vi "Event handler-Time series.vi"() -> (0 "error out":errorcluster)   [LabVIEW 2017]
uses:
  Typedefs/Read Write Enum.ctl
  Global Variables/General Globals.vi
  Global Variables/gl_UI Ctrl Refs.vi
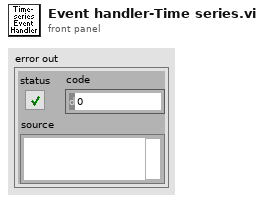
[diagram p1: front panel]
types:
  T1 = enum8{"Enabled", "Disabled", "Disabled and Grayed Out"}
  T2 = typedef "Read Write Enum.ctl" = enum16{"Read", "Write"}
  T3 = typedef "UI ctrl refs cluster.ctl" = cluster{"Top level VI path":path, "Top level VI ref":refnum<vi>, "User menu ref":refnum<k9>, "Sub Panel control":refnum<vi>, "Imaging Param Tab":refnum<vi>, "Occurrence-Start drivers":refnum<k4>, "Occurrence-Speed logging initialised":refnum<k4>, "Occurrence-XYZ stage initialised":refnum<k4>, "Exit button":refnum<vi>, "Status ind":refnum<vi>, "Set as origin":refnum<vi>, "Speed Logging":refnum<vi>, "Time Lapse":refnum<vi>, "Live Imaging":refnum<vi>, "AOL Z Stack":refnum<vi>, "Motor Z Stack":refnum<vi>, "Funct Acq button":refnum<vi>, "Hard Shutter":refnum<vi>, "Virtual Shutter":refnum<vi>, "Laser Power":refnum<vi>, "AOL Mode":refnum<vi>, "Frame Size":refnum<vi>, "Field of View":refnum<vi>, "Dwell Time":refnum<vi>, "Zoom":refnum<vi>, "AOL Z":refnum<vi>, "Objective":refnum<vi>, "Axis":refnum<vi>, "Paths & Names":refnum<vi>, "Experiment folder path (ind.)":refnum<vi>, "Last State (Ind.)":refnum<vi>, "Laser wavelength ind (nm)":refnum<vi>, "Averages":refnum<vi>, "Angle (degrees)":refnum<vi>, "X centre":refnum<vi>, "Y centre":refnum<vi>, "Plane Mode":refnum<vi>, "# Planes":refnum<vi>, "Z Start":refnum<vi>, "Z Stop":refnum<vi>, "Z Step":refnum<vi>, "PMT 1":refnum<vi>, "PMT 2":refnum<vi>, "Stage XYZ Position":refnum<vi>, "Pockels@Z Start":refnum<vi>, "Pockels@Z Stop":refnum<vi>, "Obtain Z Start":refnum<vi>, "Obtain Z Stop":refnum<vi>, "Live stim.trig.period":refnum<vi>, "Live stim.trig.enable":refnum<vi>, "Movement Correction":refnum<vi>, "Load Reference Image":refnum<vi>, "XY Stage Move":refnum<vi>, "MovCor Cluster":refnum<vi>, "RefDAQParam":refnum<vi>, "Funct. Acq. Pockels Modulation":refnum<vi>, "Background MovCor":refnum<vi>, "Ref Laser Power":refnum<vi>, "Enable Video Recording":refnum<vi>, "Video Record-Live Imaging":refnum<vi>, "Video Record-Funct acq":refnum<vi>, "Reference Source":refnum<vi>, "AOL Z-stack Chirps Ready (ind)":refnum<vi>, "Target time between mov.cor. ref triggers (ms)":refnum<vi>, "Funct. Acq. Ref frame save":refnum<vi>, "Tracking button":refnum<vi>, "Show ref plots window":refnum<vi>, "Center freq ind (nm)":refnum<vi>, "Pickup mode (ind)":refnum<vi>, "Logging queue (ind)":refnum<vi>, "Back aperture power (ind.)":refnum<vi>, "Power after objective (ind.)":refnum<vi>, "Switch user":refnum<vi>}
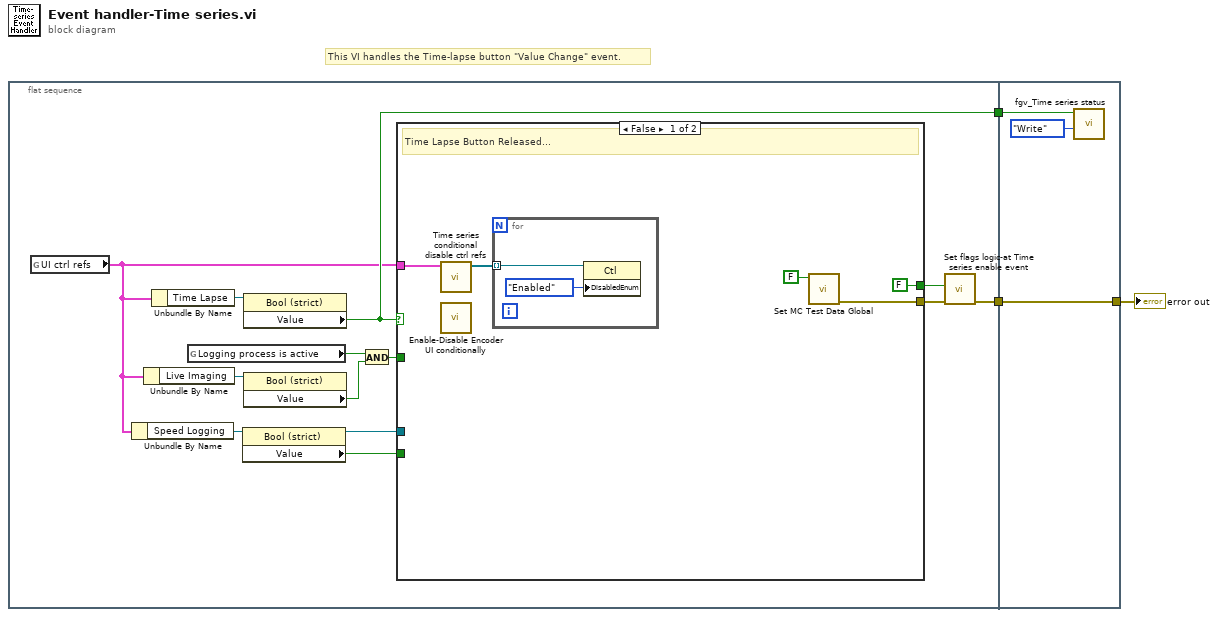
[diagram p0: block diagram]
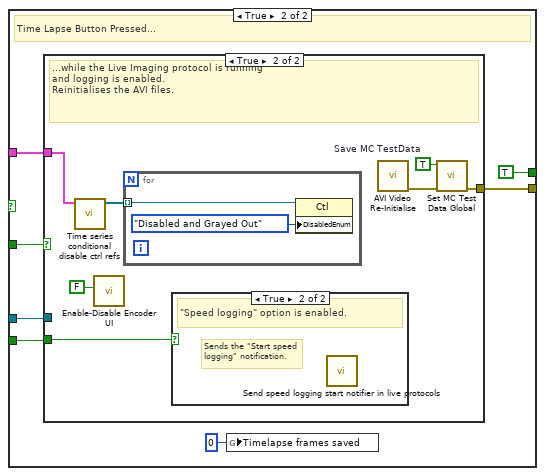
[diagram p2: hidden frame]
diagram:
  # "This VI handles the Time-lapse button \"Value Change\" event."
  n1 = flat-sequence {
    tunnel: [w5] -> w3
    tunnel: [w9] -> w2
    tunnel: [w42] -> w1
    tunnel: w3 -> [w42]
    tunnel: w2 -> [w40]
    frame #0 {
      n2 = global read "gl_UI Ctrl Refs.vi" "UI ctrl refs"() -> (w7:T3)
      n3 = Unbundle By Name(w7) -> ("Speed Logging"=w14:refnum<vi>)
      n4 = Unbundle By Name(w7) -> ("Live Imaging"=w12:refnum<vi>)
      n5 = Unbundle By Name(w7) -> ("Time Lapse"=w10:refnum<vi>)
      n6 = global read "General Globals.vi" "Logging process is active"() -> (w16:bool)
      n7 = property class="Bool (strict)"(reference=w14) -> (reference out=w8:refnum<vi>, "Value"=w13:bool)  [unwired: 1 in, 1 out]
      n8 = property class="Bool (strict)"(reference=w10) -> ("Value"=w9:bool)  [unwired: 1 in, 2 out]
      n9 = property class="Bool (strict)"(reference=w12) -> ("Value"=w11:bool)  [unwired: 1 in, 2 out]
      n10 = And(x=w16, y=w11) -> (x .and. y?=w15:bool)
      n11 = case shown="False" w9 {
        tunnel: [w20 w30] -> w4
        tunnel: w15 -> [_ w29]
        tunnel: w13 -> [_ w28]
        tunnel: w8 -> [_ w27]
        tunnel: w7 -> [w21 w26]
        tunnel: [FALSE TRUE] -> w6
        frame False {
          # "Time Lapse Button Released..."
          n12 = call "Time series conditional disable ctrl refs.vi"("UI ctrl refs"=w21) -> ("Ctrl refs"=w18:refnum<vi>[])  [unwired: 10 in]
          n13 = call "Enable-Disable Encoder UI conditionally.vi"() -> ()  [unwired: 11 in, 1 out]
          n14 = for {
            tunnel: w18 -> [w22] mode=indexing
            n15 = property class="Ctl"(reference=w22, "DisabledEnum"=T1."Enabled" ("Disabled")) -> ()  [unwired: 1 in, 2 out]
          }
          n16 = call "Set MC Test Data Global.vi"("Save MC TestData"=FALSE) -> ("error out"=w20:errorcluster)  [unwired: 10 in]
        }
        frame True {
          # "Time Lapse Button Pressed..."
          n17 = case shown="True" w29 {
            tunnel: [_ w32] -> w30
            tunnel: w28 -> [_ w37]
            tunnel: w27 -> [_ _]
            tunnel: w26 -> [_ w35]
            frame False {
              # "... while live imaging is not running \nor logging is disabled."
            }
            frame True {
              w34 = TRUE  # Save MC TestData
              # "...while the Live Imaging protocol is running \nand logging is enabled.\nReinitialises the AVI files."
              n18 = call "Time series conditional disable ctrl refs.vi"("UI ctrl refs"=w35) -> ("Ctrl refs"=w36:refnum<vi>[])  [unwired: 10 in]
              n19 = call "Enable-Disable Encoder UI.vi"("Cam VidRec.VidRec available"=FALSE) -> ()  [unwired: 10 in, 1 out]
              n20 = for {
                tunnel: w36 -> [w39] mode=indexing
                n21 = property class="Ctl"(reference=w39, "DisabledEnum"=T1."Disabled and Grayed Out" ("Disabled")) -> ()  [unwired: 1 in, 2 out]
              }
              n22 = case shown="True" w37 {
                frame False {
                  # "\"Speed logging\" option is not enabled."
                }
                frame True {
                  # "Sends the \"Start speed logging\" notification."
                  # "\"Speed logging\" option is enabled."
                  n23 = call "Send speed logging start notifier in live protocols.vi"() -> ()  [unwired: 12 in]
                }
              }
              n24 = call "AVI Video Re-Initialise.vi"() -> ("error out"=w33:errorcluster)  [unwired: 11 in]
              n25 = call "Set MC Test Data Global.vi"("error in (no error)"=w33, "Save MC TestData"=w34) -> ("error out"=w32:errorcluster)  [unwired: 9 in]
            }
          }
          n26 = global write "General Globals.vi" "Timelapse frames saved"(u32 0 ("Timelapse frames saved")) -> ()
        }
      }
      n27 = call "Set flags logic-at Time series enable event.vi"("error in (no error)"=w4, "Flag DO state"=w6) -> ("error out"=w5:errorcluster)  [unwired: 9 in]
    }
    frame #1 {
      n28 = call "fgv_Time series status.vi"("Function"=Read_Write_Enum."Write", "Timelapse?"=w40) -> ()  [unwired: 9 in, 1 out]
    }
  }
  "error out" <- w1
